vi "Go SSARA.vi"() -> ()   [LabVIEW 2016]
uses:
  <vilib>/Platform/TimedLoop/XDataNode/timing_clust.ctl
  <vilib>/Platform/TimedLoop/XDataNode/nitl_modes.ctl
  <vilib>/Platform/TimedLoop/XDataNode/wakeup.ctl
  <vilib>/Simulation/Scripting/Companion Diagram/SimConfigNode/SimParams.ctl
  <vilib>/Simulation/Scripting/Companion Diagram/SimConfigNode/_simSolvers.ctl
  <vilib>/Simulation/Implementation/Shared/SIMSCR Execution Mode.ctl
  <vilib>/Simulation/Param Hierarchy/Typedefs/SIMPH Param Control Actions.ctl
  <vilib>/Simulation/Scripting/Editor Utilities/SIM subVI tag data.ctl
  <vilib>/Simulation/Scripting/Editor Utilities/SIM subVI execution type.ctl
  <vilib>/Simulation/Implementation/Shared/NILVSim_ParamChanged.vi
  <vilib>/Simulation/Implementation/Shared/NILVSim_FinishedLate.vi
  <vilib>/Simulation/Implementation/Shared/NILVSIM_BeginStep.vi
  <vilib>/Simulation/SignalDisplay/Implementation/NILVSim Buffer XY Graph.llb/SIM Buffer XY Graph (scalar).vi
  <vilib>/Simulation/Implementation/Shared/SIM Fire Discrete SubVI.vi
  <vilib>/Simulation/Implementation/Shared/NILVSim_Manager.vi
  <vilib>/Utility/error.llb/Clear Errors.vi
  <vilib>/Simulation/Implementation/Shared/NILVSim_FinalizeModel.vi
  <vilib>/Simulation/SignalDisplay/Implementation/NILVSim Buffer XY Graph.llb/NILVSim Buffer XY Graph (core).vi
  <vilib>/Simulation/Implementation/Shared/SIM manage modulo counter.vi
  <vilib>/Simulation/Implementation/Shared/SIM Circular Buffer.llb/SIM CircBuf remove oldest.vi
  <vilib>/Simulation/Implementation/Shared/SIM Circular Buffer.llb/SIM circular buffer insert.vi
  <vilib>/Simulation/Implementation/Shared/SIM Fire Discrete SubVI (Core).vi
  <vilib>/Simulation/Implementation/Shared/SIM Unbundle Sim Info.vi
  <vilib>/Simulation/Implementation/Shared/SIMSH Read Queue.vi
  <vilib>/Simulation/Implementation/Shared/NILVSim_Initialize.vi
  <vilib>/Simulation/Utility/Implementation/NILVSim Get Time and IsAcceptedStep.vi
  <vilib>/Simulation/Implementation/Shared/SIM Circular Buffer.llb/SIM circular buffer create.vi
  <vilib>/Simulation/Implementation/Shared/SIM Circular Buffer.llb/SIM circular buffer ordered array.vi
  <vilib>/Simulation/Implementation/Shared/NILVSim_GetModelError.vi
  <vilib>/Simulation/Implementation/Shared/SIM Bundle Sim Info.vi
  <vilib>/Platform/TimedLoop/XDataNode/XDataNode.xnode
  <vilib>/Simulation/Scripting/Companion Diagram/SimConfigNode/SimDog.xnode
  <vilib>/Simulation/Implementation/XNodeFramework/SimXNode/SimX.xnode
  <vilib>/Platform/TimedLoop/XDataNode/XDNodeRunTimeDep.lvlib
  <vilib>/Simulation/Implementation/Shared/NI_SIM_Implementation.lvlib
panel:
  in  "탭 컨트롤":T1(tab)
  out "x_Nav KF":dbl format="%#.8g"
  out "y_Nav KF":dbl format="%#.8g"
  out "x_Nav Raw":dbl format="%#.8g"
  out "y_Nav Raw":dbl format="%#.8g"
  out "Checksum":bool
  out "Valid":bool
  out "GPS_Speed":dbl
  out "GPS_Longitude":dbl
  out "GPS_Latitude":dbl
  out "GPS_Heading angle":dbl
  out "IMU_Yaw":dbl
  out "Encoder Speed":dbl
  out "x_EKF":dbl
  out "y_EKF":dbl
  out "Heading_EKF":dbl
  out "Speed_EKF":dbl
  out "Vision Lane":dbl[][](array[numeric])
  out "Lidar Obstacle":dbl[][](array[numeric])
  out "Platform Data":u16[](array[numeric])
  out "IMU_Roll":dbl
  out "IMU_Pitch":dbl
  out "IMU_Acceleration":dbl
  out "Total Distance":dbl
  out "ALIVE":u16
  in  "SPEED":u16
  in  "STEER":u16
  in  "GEAR":u16(ring) items=["Forward Drive", "Neutral", "Backward Drive"]
  in  "A or M":bool
  in  "BRAKE":u16
  in  "Platform_E-STOP":bool
  in  "Event":T2(ring)
  out "EKF Nav":T3(graph)
  out "KF Nav":T3(graph)
  in  "EKF_Q (시스템 잡음)":dbl[][](array[numeric])=[[50000.0, 0.0, 0.0, 0.0], [0.0, 50000.0, 0.0, 0.0], [0.0, 0.0, 0.001, 0.0], [0.0, 0.0, 0.0, 0.01]]
  in  "EKF_R (측정 잡음)":dbl[][](array[numeric])=[[100000000.0, 0.0, 0.0, 0.0], [0.0, 100000000.0, 0.0, 0.0], [0.0, 0.0, 100000.0, 0.0], [0.0, 0.0, 0.0, 10.0]]
  in  "KF_R (측정 잡음)":dbl[][](array[numeric])=[[1e-05, 0.0], [0.0, 1e-05]]
  in  "KF_Q (시스템 잡음)":dbl[][](array[numeric])=[[0.001, 0.0], [0.0, 0.001]]
  out "Heading Angle":T4(graph)
  in  "위도경도 Raw":path=path "C:/Users/user/Desktop/[Github]_GPS Team/데이터/GPS Raw.txt"
  in  "GPS port num":refnum<visa-resource-name>="COM9"
  in  "IMU port num":refnum<visa-resource-name>="COM3"
  in  "LIDAR Address":string="192.168.0.204"
  in  "LIDAR port num":u16=2111
  in  "Platform port in":refnum<visa-resource-name>="COM4"
  out "End Loop":bool=TRUE
  # "GPS Data"
  # "IMU, Encoder Data"
  # "KF Data"
  # "EKF Data"
  # "VISION Lane"
  # "LIDAR Obstacle"
  # "Platform Data"
  # "Port Setting"
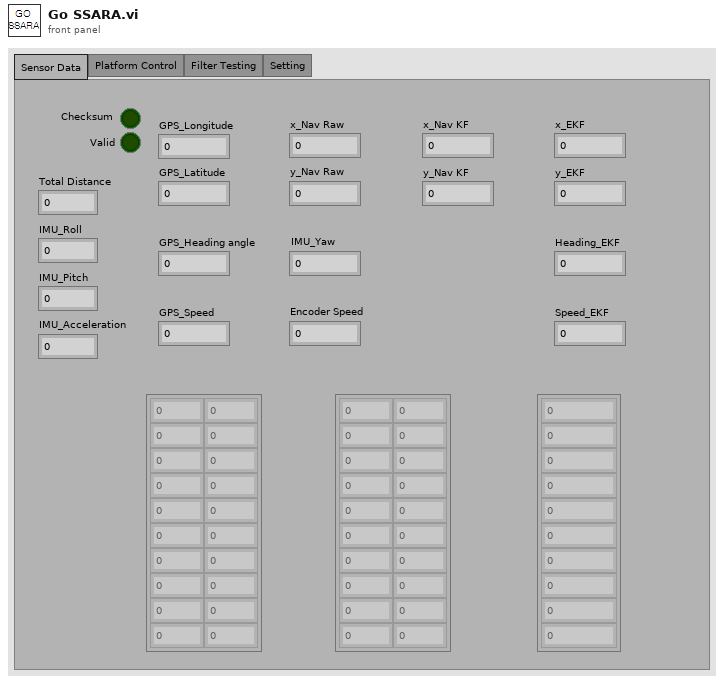
[diagram p1: front panel]
types:
  T1 = enum32{"Sensor Data", "Platform Control", "Filter Testing", "Setting"}
  T2 = enum16{"기본", "횡단보도", "협로주행", "정적 장애물", "동적 장애물", "유턴", "주차"}
  T3 = cluster{"XY Graph":cluster{"X":dbl, "Y":dbl}[]}[]
  T4 = cluster{"GPS Raw_Heading angle":dbl, "IMU_Yaw":dbl}
  T5 = typedef "XDNodeRunTimeDep.lvlib/timing_clust.ctl" = cluster{"Expected End [f-1]":u64, "Actual End [f-1]":u64, "Finished Late? [f-1]":bool, "Expected End [i-1]":u64, "Actual End [i-1]":u64, "Finished Late? [i-1]":bool, "Expected Start [i]":u64, "Actual Start [i]":u64, "Expected Start [f]":u64, "Actual Start [f]":u64, "Source Name":string, "Structure Name":string, "Period":i64, "Deadline":i64, "Offset":i64, "Start":i64, "Priority":i32, "Timeout":i32, "Mode":T6, "Wakeup Reason":T7, "Error":errorcluster, "Source Type":string, "Secondary Source Type":string, "Global End Time":u64, "Global Start Time":u64, "Frame Duration":u64, "Iteration Duration":u64, "Assigned CPU":i32, "I/O Scan Engine Mode":u32}
  T6 = typedef "XDNodeRunTimeDep.lvlib/nitl_modes.ctl" = enum32{"No Change", "Process missed periods, maintain original phase", "Discard missed periods, maintain original phase", "Process missed periods, ignore original phase", "Discard missed periods, ignore original phase"}
  T7 = typedef "XDNodeRunTimeDep.lvlib/wakeup.ctl" = enum32{"Normal", "Aborted", "Asynchronous wakeup", "Timing source error", "Timed loop error", "Timeout"}
  T8 = typedef "SIMSCR Execution Mode.ctl" = enum16{"Simulate to Completion", "Single Time-Step Simulation (Fixed Step Only)"}
  T9 = typedef "SIMPH Param Control Actions.ctl" = enum16{"get params", "set params"}
  T10 = typedef "SIM subVI tag data.ctl" = cluster{"period":dbl, "skew":dbl, "Simulation execution type":T11}
  T11 = typedef "SIM subVI execution type.ctl" = enum16{"Function call", "Discrete", "Continuous", "Initialization only", "Final step only"}
  T12 = typedef "SimParams.ctl" = cluster{"Initial Time (s)":dbl, "Final Time (s)":dbl, "Step Size (s)":dbl, "ODE Solver":T13, "Minimum Step Size (s)":dbl, "Maximum Step Size (s)":dbl, "Relative Tolerance":dbl, "Absolute Tolerance":dbl, "Software Timing":bool, "Initial Step Size (s)":dbl, "Automatic Fixed Step Size?":bool, "Automatic Discrete Step Size?":bool, "Discrete Step Size (s)":dbl, "Calculate using Time Step":bool, "Solver Wired?":bool, "Prev.Frm.Expected End":u64, "Prev.Frm.Actual End":u64, "Prev.Frm.Finished Late?":bool, "Prev.Iter.Expected End":u64, "Prev.Iter.Actual End":u64, "Prev.Iter.Finished Late?":bool, "Expected Iteration Start":u64, "Actual Iteration Start":u64, "Expected Frame Start":u64, "Actual Frame Start":u64, "Source Name":string, "Name":string, "Period":i64, "Deadline":i64, "Offset":i64, "Start":i64, "Priority":i32, "Timeout":i32, "Processor":i32, "Mode":enum32{"No Change", "Process missed periods, maintain original phase", "Discard missed periods, maintain original phase", "Process missed periods, ignore original phase", "Discard missed periods, ignore original phase"}, "Wakeup reason":enum32{"Normal", "Aborted", "Asynchronous wakeup", "Timing source error", "Timed loop error", "Timeout"}, "Error":errorcluster, "Source Type":string, "Secondary Source Type":string, "Global End Time":u64, "Global Start Time":u64, "Full Solver Reset":bool, "Execution Mode":T8, "Nan/Inf Check":bool, "Custom Solver Library":string, "Solver Is Variable":bool, "custom solver name":string, "Signal Collection Decimation":u32}
  T13 = typedef "_simSolvers.ctl" = enum16{"Runge-Kutta 1 (Euler)", "Runge-Kutta 2", "Runge-Kutta 3", "Runge-Kutta 4", "Runge-Kutta 23 (variable)", "Runge-Kutta 45 (variable)", "BDF (variable)", "Adams-Moulton (variable)", "Rosenbrock (variable)", "Discrete States Only", "SDIRK 4 (variable)", "Radau 5 (variable)", "Radau 9 (variable)", "Radau 13 (variable)", "Radau [Variable Order] (variable)", "Gear's Method (variable)", "Linearizer", "State Query", "Trim Eval", "Custom Solver"}
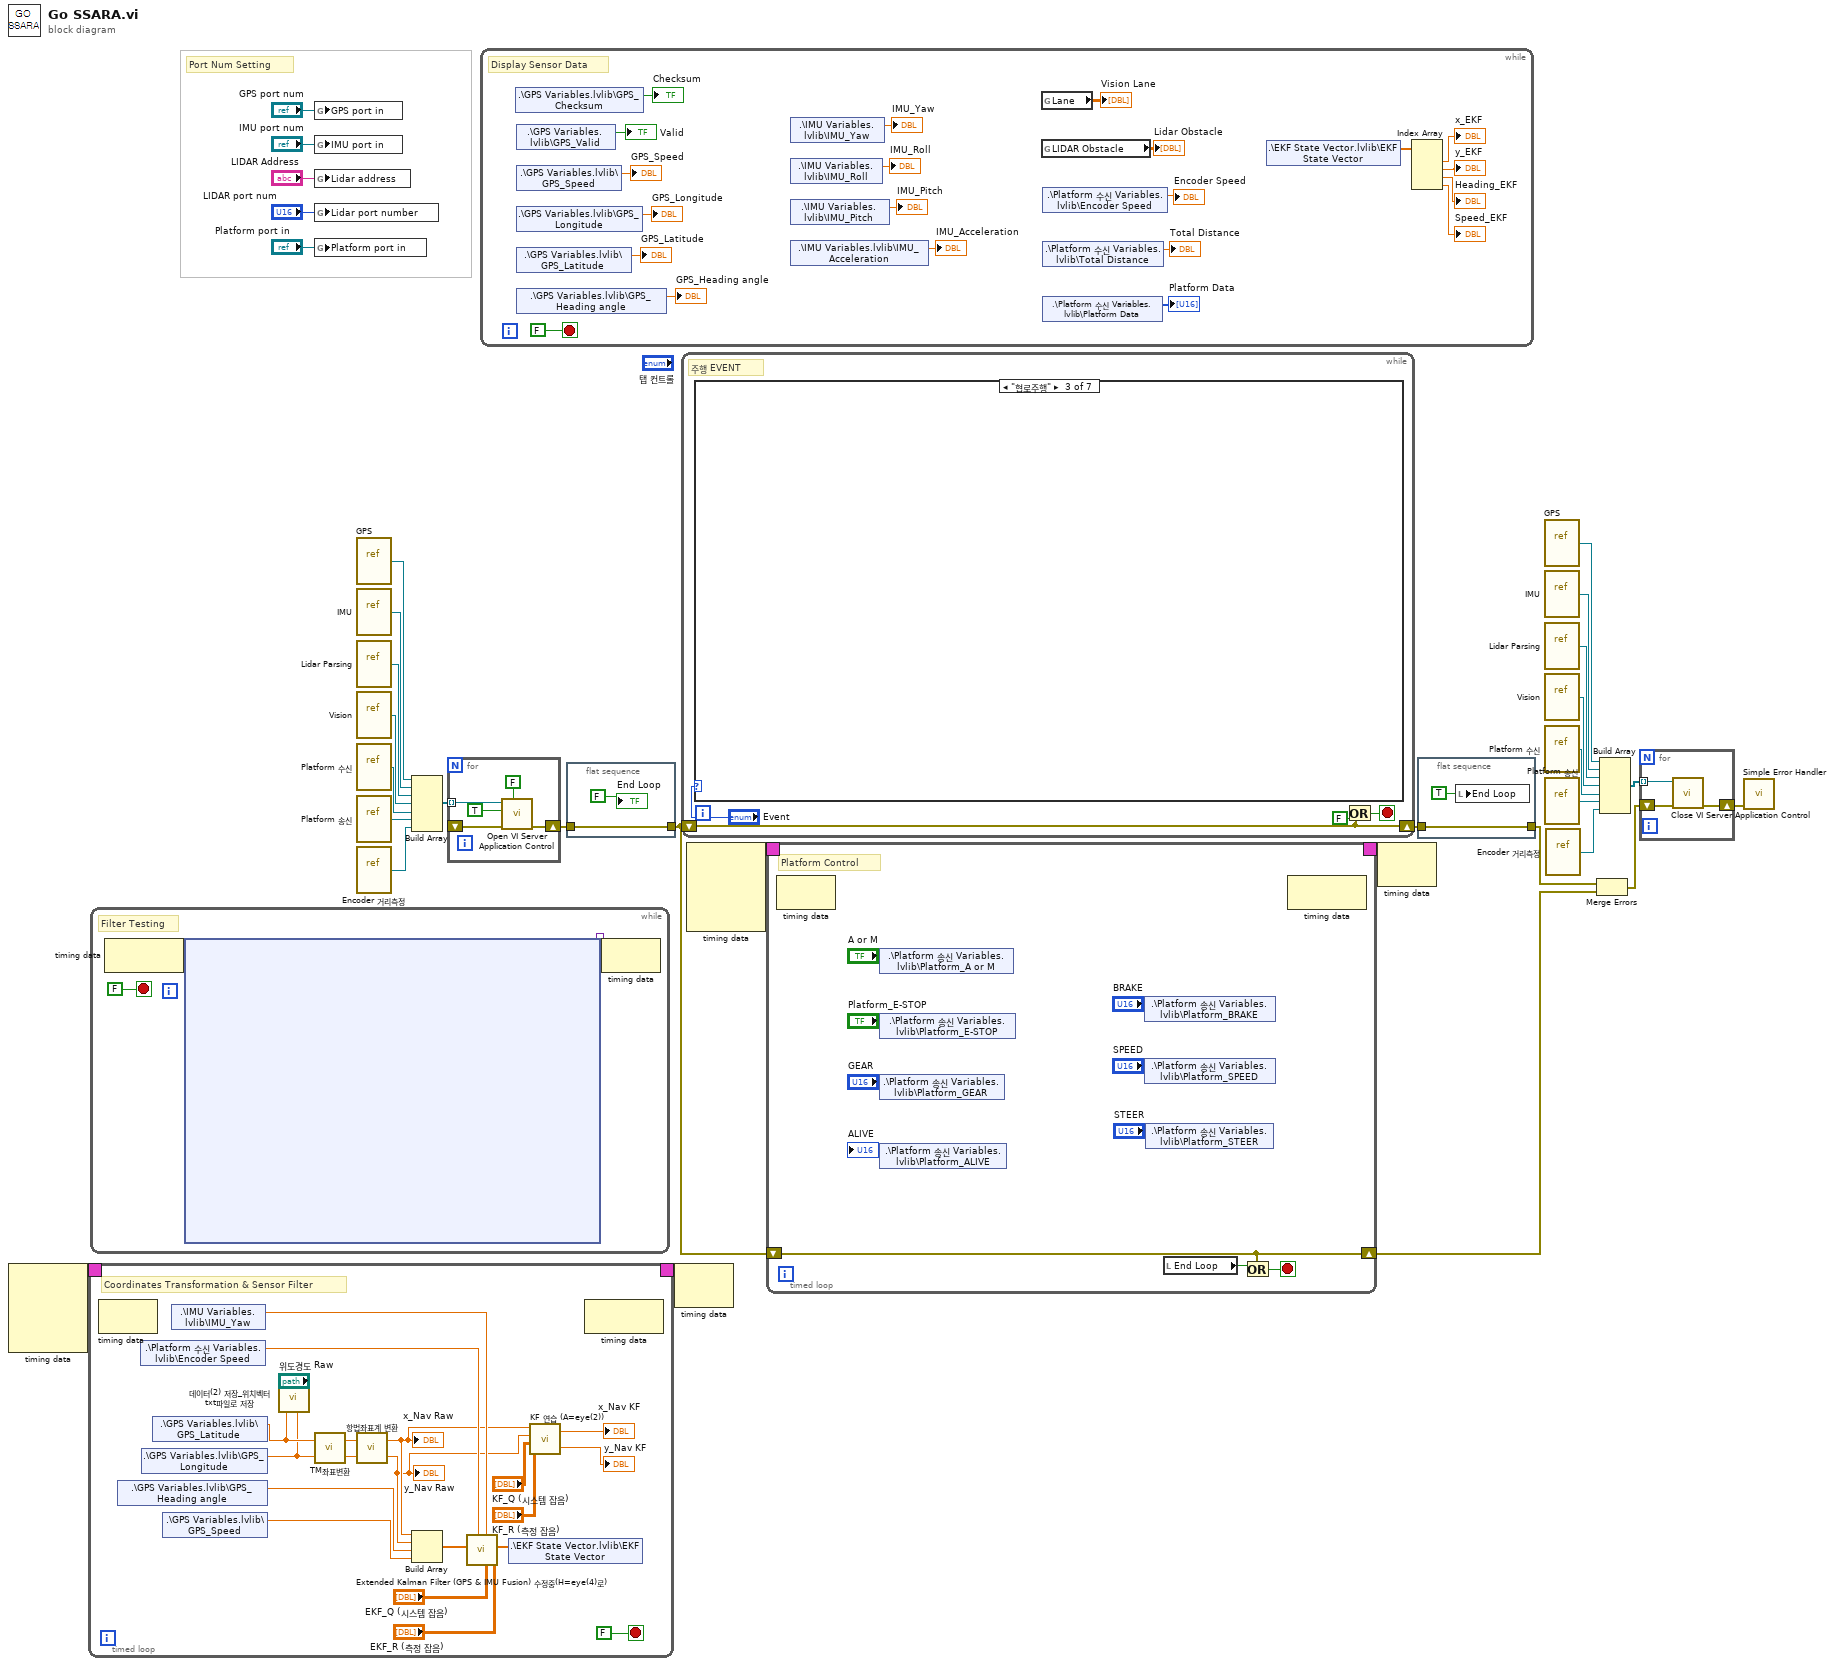
[diagram p0: block diagram]
diagram:
  # "Port Num Setting"
  n1 = node-c288() -> (w4:T5)  [unwired: 4 in]
  n2 = timed-loop {
    timing: w4 -> [_]
    timing-out: [_] -> w3
    stop <- FALSE stop-if-true
    # "Coordinates Transformation & Sensor Filter"
    n3 = node-c288() -> ()  [unwired: 1 in, 1 out]
    n4 = shared-variable ".\\GPS Variables.lvlib\\GPS_Heading angle"() -> (w49:dbl)  [unwired: 1 in, 1 out]
    n5 = shared-variable ".\\Platform 수신 Variables.lvlib\\Encoder Speed"() -> (w43:dbl)  [unwired: 1 in, 1 out]
    n6 = shared-variable ".\\GPS Variables.lvlib\\GPS_Longitude"() -> (w39:dbl)  [unwired: 1 in, 1 out]
    n7 = shared-variable ".\\GPS Variables.lvlib\\GPS_Latitude"() -> (w40:dbl)  [unwired: 1 in, 1 out]
    n8 = shared-variable ".\\GPS Variables.lvlib\\GPS_Speed"() -> (w48:dbl)  [unwired: 1 in, 1 out]
    n9 = shared-variable ".\\IMU Variables.lvlib\\IMU_Yaw"() -> (w42:dbl)  [unwired: 1 in, 1 out]
    n10 = call "데이터(2) 저장_위치벡터  txt파일로 저장.vi"("Location"="위도경도 Raw", "Data2"=w39, "Data1"=w40) -> ()
    n11 = call "TM좌표변환.vi"("lon"=w39, "lat"=w40) -> ("Y_TM"=w50:dbl, "X_TM"=w51:dbl)
    n12 = call "항법좌표계 변환.vi"("Y_TM"=w50, "X_TM"=w51) -> ("Y_Nav"=w37:dbl, "X_Nav"=w38:dbl)
    "x_Nav Raw" <- w38
    "y_Nav Raw" <- w37
    n13 = Build Array(w38, w37, w49, w48) -> (w47:dbl[])
    n14 = call "Extended Kalman Filter (GPS & IMU Fusion) 수정중(H=eye(4)로).vi"("R (v의 공분산행렬_측정잡음)_모델링필요"="EKF_R (측정 잡음)", "Q (w의 공분산행렬_시스템잡음)_모델링필요"="EKF_Q (시스템 잡음)", "theta_IMU"=w42, "v_Encoder"=w43, "X_GPS Raw"=w47) -> ("X_EKF"=w46:dbl[])  [unwired: 6 in]
    n15 = shared-variable ".\\EKF State Vector.lvlib\\EKF State Vector"(w46) -> ()  [unwired: 1 in, 1 out]
    n16 = call "KF 연습 (A=eye(2)).vi"("R"="KF_R (측정 잡음)", "Q"="KF_Q (시스템 잡음)", "Y_input"=w37, "X_input"=w38) -> ("Y_Filtered"=→"y_Nav KF":dbl, "X_Filtered"=→"x_Nav KF":dbl)
    n17 = node-c288() -> ()  [unwired: 1 in, 1 out]
  }
  n18 = while {
    stop <- FALSE stop-if-true
    # "Filter Testing"
    n19 = node-c288() -> (w56:variant)  [unwired: 1 out]
    n20 = node-c254 ("Simulation Loop")(w56) -> (w55:variant)
    n21 = node-c288(w55) -> ()  [unwired: 1 out]
  }
  n22 = global write "[GV]_GPS Port NUM.vi" "GPS port in"("GPS port num") -> ()
  n23 = global write "[GV]_IMU Port NUM.vi" "IMU port in"("IMU port num") -> ()
  n24 = global write "[GV]_LIDAR Ethernet Address.vi" "Lidar address"("LIDAR Address") -> ()
  n25 = global write "[GV]_LIDAR Port NUM.vi" "Lidar port number"("LIDAR port num") -> ()
  n26 = global write "[GV]_PLATFORM Port NUM.vi" "Platform port in"("Platform port in") -> ()
  n27 = vi-ref "GPS.vi"() -> (w23:refnum<vi>)
  n28 = vi-ref "IMU.vi"() -> (w22:refnum<vi>)
  n29 = vi-ref "Lidar Parsing.vi"() -> (w21:refnum<vi>)
  n30 = vi-ref "Vision.vi"() -> (w20:refnum<vi>)
  n31 = vi-ref "Platform 수신.vi"() -> (w19:refnum<vi>)
  n32 = vi-ref "Platform 송신.vi"() -> (w18:refnum<vi>)
  n33 = vi-ref "Encoder 거리측정.vi"() -> (w2:refnum<vi>)
  n34 = Build Array(w23, w22, w21, w20, w19, w18, w2) -> (w17:refnum<vi>[])
  n35 = for {
    tunnel: w17 -> [w469] mode=indexing
    shift-right: [w466] -> w29
    shift-left: _ -> [w465]
    n36 = call "Open VI Server Application Control.vi"("open front panel (F)"=FALSE ("Open Front Panel"), "error in (no error)"=w465, "run VI (F)"=TRUE ("Run VI"), "VI refnum"=w469) -> ("error out"=w466:errorcluster)  [unwired: 7 in]
  }
  n37 = while {
    stop <- FALSE stop-if-true
    # "Display Sensor Data"
    n38 = shared-variable ".\\GPS Variables.lvlib\\GPS_Checksum"() -> (→"Checksum":bool)  [unwired: 1 in, 1 out]
    n39 = shared-variable ".\\GPS Variables.lvlib\\GPS_Valid"() -> (→"Valid":bool)  [unwired: 1 in, 1 out]
    n40 = shared-variable ".\\GPS Variables.lvlib\\GPS_Speed"() -> (→"GPS_Speed":dbl)  [unwired: 1 in, 1 out]
    n41 = shared-variable ".\\GPS Variables.lvlib\\GPS_Longitude"() -> (→"GPS_Longitude":dbl)  [unwired: 1 in, 1 out]
    n42 = shared-variable ".\\GPS Variables.lvlib\\GPS_Latitude"() -> (→"GPS_Latitude":dbl)  [unwired: 1 in, 1 out]
    n43 = shared-variable ".\\GPS Variables.lvlib\\GPS_Heading angle"() -> (→"GPS_Heading angle":dbl)  [unwired: 1 in, 1 out]
    n44 = shared-variable ".\\IMU Variables.lvlib\\IMU_Yaw"() -> (→"IMU_Yaw":dbl)  [unwired: 1 in, 1 out]
    n45 = shared-variable ".\\IMU Variables.lvlib\\IMU_Roll"() -> (→"IMU_Roll":dbl)  [unwired: 1 in, 1 out]
    n46 = shared-variable ".\\IMU Variables.lvlib\\IMU_Pitch"() -> (→"IMU_Pitch":dbl)  [unwired: 1 in, 1 out]
    n47 = shared-variable ".\\IMU Variables.lvlib\\IMU_Acceleration"() -> (→"IMU_Acceleration":dbl)  [unwired: 1 in, 1 out]
    n48 = global read "[GV]_Vision Lane.vi" "Lane"() -> (→"Vision Lane":dbl[][])
    n49 = global read "[GV]_Lidar Obstacle.vi" "LIDAR Obstacle"() -> (→"Lidar Obstacle":dbl[][])
    n50 = shared-variable ".\\Platform 수신 Variables.lvlib\\Encoder Speed"() -> (→"Encoder Speed":dbl)  [unwired: 1 in, 1 out]
    n51 = shared-variable ".\\Platform 수신 Variables.lvlib\\Total Distance"() -> (→"Total Distance":dbl)  [unwired: 1 in, 1 out]
    n52 = shared-variable ".\\Platform 수신 Variables.lvlib\\Platform Data"() -> (→"Platform Data":u16[])  [unwired: 1 in, 1 out]
    n53 = shared-variable ".\\EKF State Vector.lvlib\\EKF State Vector"() -> (w475:dbl[])  [unwired: 1 in, 1 out]
    n54 = Index Array(array=w475) -> (element #1=→"x_EKF":dbl, element #2=→"y_EKF":dbl, element #3=→"Heading_EKF":dbl, element #4=→"Speed_EKF":dbl)  [unwired: 4 in]
  }
  n55 = flat-sequence {
    tunnel: w29 -> [w491]
    tunnel: [w491] -> w27
    frame #0 {
      "End Loop" <- FALSE ("Halt TL")
    }
  }
  n56 = node-c288(w3) -> ()  [unwired: 1 out]
  n57 = while {
    shift-right: [w494] -> w28
    shift-left: w27 -> [w494]
    stop <- w495 stop-if-true
    # "주행 EVENT"
    n58 = case shown="\"협로주행\"" "Event" {
      frame "기본", Default {
      }
      frame "횡단보도" {
      }
      frame "협로주행" {
      }
      frame "정적 장애물" {
      }
      frame "동적 장애물" {
      }
      frame "유턴" {
      }
      frame "주차" {
      }
    }
    n59 = Or(x=w494, y=FALSE) -> (x .or. y?=w495:bool)
  }
  n60 = node-c288() -> (w31:T5)  [unwired: 4 in]
  n61 = timed-loop {
    timing: w31 -> [_]
    timing-out: [_] -> w30
    shift-right: [w505] -> w25
    shift-left: w27 -> [w505]
    stop <- w506 stop-if-true
    # "Platform Control"
    n62 = node-c288() -> ()  [unwired: 1 in, 1 out]
    n63 = shared-variable ".\\Platform 송신 Variables.lvlib\\Platform_A or M"("A or M") -> ()  [unwired: 1 in, 1 out]
    n64 = shared-variable ".\\Platform 송신 Variables.lvlib\\Platform_E-STOP"("Platform_E-STOP") -> ()  [unwired: 1 in, 1 out]
    n65 = shared-variable ".\\Platform 송신 Variables.lvlib\\Platform_GEAR"("GEAR") -> ()  [unwired: 1 in, 1 out]
    n66 = shared-variable ".\\Platform 송신 Variables.lvlib\\Platform_ALIVE"() -> (→"ALIVE":u16)  [unwired: 1 in, 1 out]
    n67 = shared-variable ".\\Platform 송신 Variables.lvlib\\Platform_BRAKE"("BRAKE") -> ()  [unwired: 1 in, 1 out]
    n68 = shared-variable ".\\Platform 송신 Variables.lvlib\\Platform_SPEED"("SPEED") -> ()  [unwired: 1 in, 1 out]
    n69 = shared-variable ".\\Platform 송신 Variables.lvlib\\Platform_STEER"("STEER") -> ()  [unwired: 1 in, 1 out]
    n70 = local read "End Loop"() -> (w504:bool)
    n71 = Or(x=w504, y=w505) -> (x .or. y?=w506:bool)
    n72 = node-c288() -> ()  [unwired: 1 in, 1 out]
  }
  n73 = node-c288(w30) -> ()  [unwired: 1 out]
  n74 = flat-sequence {
    tunnel: w28 -> [w510]
    tunnel: [w510] -> w26
    frame #0 {
      n75 = local write "End Loop"(TRUE ("End Loop")) -> ()
    }
  }
  n76 = vi-ref "GPS.vi"() -> (w16:refnum<vi>)
  n77 = vi-ref "IMU.vi"() -> (w15:refnum<vi>)
  n78 = vi-ref "Lidar Parsing.vi"() -> (w14:refnum<vi>)
  n79 = vi-ref "Vision.vi"() -> (w13:refnum<vi>)
  n80 = vi-ref "Platform 수신.vi"() -> (w12:refnum<vi>)
  n81 = vi-ref "Platform 송신.vi"() -> (w11:refnum<vi>)
  n82 = vi-ref "Encoder 거리측정.vi"() -> (w1:refnum<vi>)
  n83 = Merge Errors(w26, w25) -> (w24:errorcluster)
  n84 = Build Array(w16, w15, w14, w13, w12, w11, w1) -> (w10:refnum<vi>[])
  n85 = for {
    tunnel: w10 -> [w511] mode=indexing
    shift-right: [w513] -> w32
    shift-left: w24 -> [w512]
    n86 = call "Close VI Server Application Control.vi"("error in (no error)"=w512, "VI refnum"=w511) -> ("error out"=w513:errorcluster)  [unwired: 9 in]
  }
  n87 = call <vilib>:"Simple Error Handler.vi"("error in (no error)"=w32) -> ()  [unwired: 4 in, 5 out]
